vi "Turn compressor and cold head ON-OFF.vi"(8 "error in":errorcluster, 10 "F-70 parameters in":T1 {"Last updated" format="%<%d/%m/%Y %H:%M:%S>T"; "State of operation" items=["Local Off", "Local On", "Remote Off", "Remote On", "Cold head Run", "Cold head pause", "Fault Off", "Oil Fault Off"]; "Return pressure (PSIG)" scale=0.0..200.0; "Water in Tmp (°C)" scale=0.0..100.0; "Water out Tmp (°C)" scale=0.0..100.0; "He discharge Tmp (°C)" scale=0.0..100.0}, 11 "VISA resource in":refnum<visa-resource-name>) -> (0 "error out":errorcluster, 1 "State of operation":u16(ring) items=["Local Off", "Local On", "Remote Off", "Remote On", "Cold head Run", "Cold head pause", "Fault Off", "Oil Fault Off"], 2 "F-70 parameters out":T1 {"Last updated" format="%<%d/%m/%Y %H:%M:%S>T"; "State of operation" items=["Local Off", "Local On", "Remote Off", "Remote On", "Cold head Run", "Cold head pause", "Fault Off", "Oil Fault Off"]; "Return pressure (PSIG)" scale=0.0..200.0; "Water in Tmp (°C)" scale=0.0..100.0; "Water out Tmp (°C)" scale=0.0..100.0; "He discharge Tmp (°C)" scale=0.0..100.0}, 3 "VISA resource out":refnum<visa-resource-name>)   [LabVIEW 2021, in "F-70 driver.lvlib"]
doc: "ON: When the compressor is off and without active fault, this will turn the compressor and\ncold head on.\nOFF: When the compressor and/or cold head is on, this will turn either or both off."
uses:
  <instrlib>/F-70 driver/F-70 driver.lvlib
  <instrlib>/F-70 driver/public/F-70 parameters.ctl
  <instrlib>/F-70 driver/public/Commands.ctl
panel:
  in  "Action (ON)":bool=TRUE
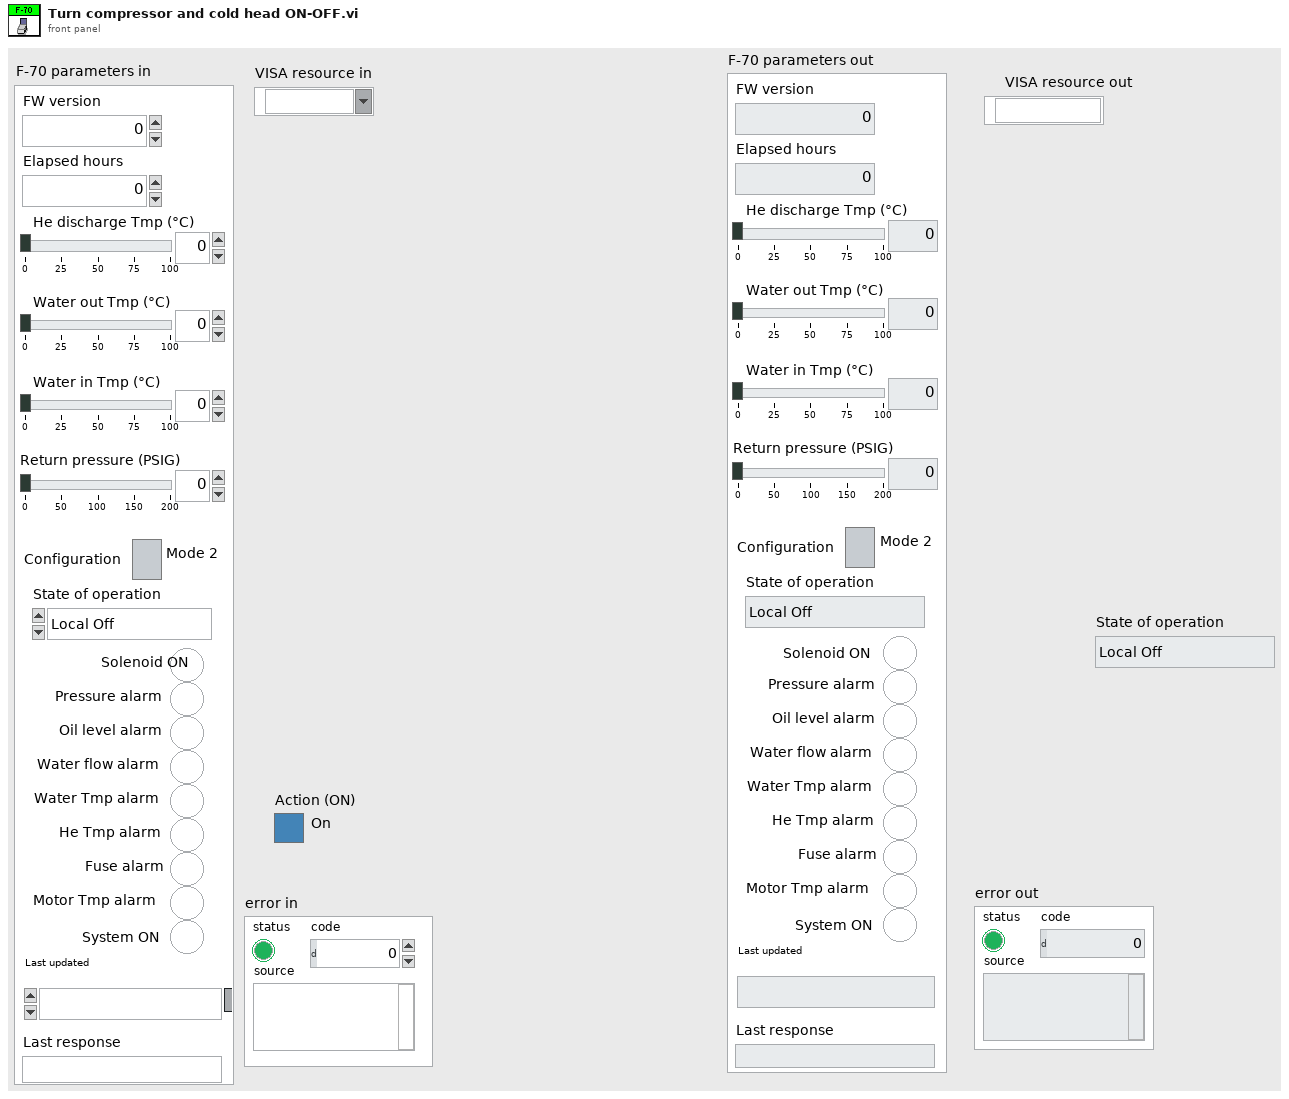
[diagram p1: front panel]
types:
  T1 = typedef "F-70 driver.lvlib/F-70 parameters.ctl" = cluster{"FW version":dbl, "Elapsed hours":dbl, "He discharge Tmp (°C)":dbl, "Water out Tmp (°C)":dbl, "Water in Tmp (°C)":dbl, "Return pressure (PSIG)":dbl, "Configuration":bool, "State of operation":u16, "Solenoid ON":bool, "Pressure alarm":bool, "Oil level alarm":bool, "Water flow alarm":bool, "Water Tmp alarm":bool, "He Tmp alarm":bool, "Fuse alarm":bool, "Motor Tmp alarm":bool, "System ON":bool, "Last updated":timestamp, "Last response":string}
  T2 = typedef "F-70 driver.lvlib/Commands.ctl" = enum16{"TEA", "PRA", "STA", "ID1", "ON1", "RS1", "CHP", "OFF", "CHR", "POF", "TE1", "TE2", "TE3", "TE4", "PR1", "PR2", "???"}
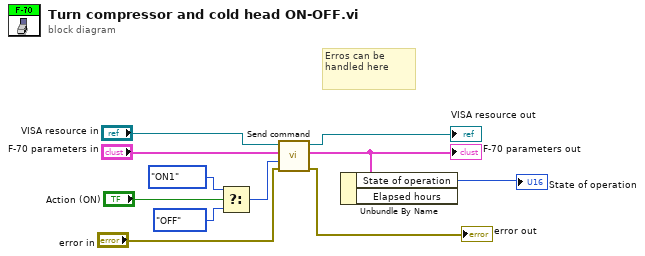
[diagram p0: block diagram]
diagram:
  # "Erros can be\nhandled here"
  n1 = Select(t=Commands."ON1" ("Array"), s="Action (ON)", f=Commands."OFF" ("Array")) -> (s? t:f=w3:T2)
  n2 = call <instrlib>:"Send command.vi"("error in"="error in", "Command"=w3, "F-70 parameters in"="F-70 parameters in", "VISA resource in"="VISA resource in") -> ("error out"=→"error out":errorcluster, "F-70 parameters in 2"=w6:T1, "VISA resource out"=→"VISA resource out":refnum<visa-resource-name>)  [unwired: 1 in]
  "F-70 parameters out" <- w6
  n3 = Unbundle By Name(w6) -> ("State of operation"=→"State of operation":u16)  [unwired: 1 out]
